vi "UniCyRO_Sim 2.vi"() -> ()   [LabVIEW 2012]
doc: "This VI starts and stops the environment simulator and serves as the master VI for your simulation code. Open and run this VI to display the environment simulator, or open the block diagram to view or modify simulation code."
uses:
  <vilib>/robotics/Simulator/Engine/ctl/Step Mode.ctl
  <vilib>/robotics/Simulator/Engine/ctl/Simulation Mode.ctl
  <vilib>/Simulation/Scripting/Companion Diagram/SimConfigNode/SimParams.ctl
  <vilib>/Simulation/Scripting/Companion Diagram/SimConfigNode/_simSolvers.ctl
  <vilib>/Simulation/Implementation/Shared/SIMSCR Execution Mode.ctl
  <vilib>/Platform/TimedLoop/XDataNode/timing_clust.ctl
  <vilib>/Platform/TimedLoop/XDataNode/nitl_modes.ctl
  <vilib>/Platform/TimedLoop/XDataNode/wakeup.ctl
  <vilib>/Simulation/Param Hierarchy/Typedefs/SIMPH Param Control Actions.ctl
  <vilib>/Simulation/Scripting/Editor Utilities/SIM subVI tag data.ctl
  <vilib>/Simulation/Scripting/Editor Utilities/SIM subVI execution type.ctl
  <vilib>/Simulation/Implementation/Shared/NILVSim_ParamChanged.vi
  <vilib>/Simulation/Implementation/Shared/NILVSim_FinishedLate.vi
  <vilib>/Simulation/Utility/Implementation/SIM Time.vi
  <vilib>/Simulation/Utility/Implementation/SIM Halt.vi
  <vilib>/Simulation/Implementation/Shared/SIM Fire Discrete SubVI.vi
  <vilib>/Simulation/Implementation/Shared/NILVSim_Manager.vi
  <vilib>/Simulation/Implementation/Shared/NILVSim_FinalizeModel.vi
  <vilib>/Simulation/Implementation/Shared/SIM Fire Discrete SubVI (Core).vi
  <vilib>/Simulation/Implementation/Shared/SIM Unbundle Sim Info.vi
  <vilib>/Utility/error.llb/Clear Errors.vi
  <vilib>/Simulation/Implementation/Shared/NILVSim_GetModelError.vi
  <vilib>/Simulation/Implementation/Shared/SIM Bundle Sim Info.vi
  <vilib>/Simulation/Implementation/Shared/SIMSH Read Queue.vi
  <vilib>/Simulation/Implementation/Shared/NILVSim_Initialize.vi
  Model/UniCyRO/Read Sensors.vi
  <vilib>/robotics/Simulator/Interface/Simulator References/Get Simulator Reference.vi
  <vilib>/robotics/Simulator/Interface/Simulator References/Get Joint Reference (Hinge).vi
  <vilib>/Simulation/Utility/Implementation/NILVSim Get Time and IsAcceptedStep.vi
  <vilib>/robotics/Simulator/Interface/Take Simulation Steps.vi
  <vilib>/Simulation/Scripting/Companion Diagram/SimConfigNode/SimDog.xnode
  Control Systems/PIDparallelController.vi
  Model/UniCyRO/UniCyRO_Host_Sim.lvclass
  <vilib>/Platform/TimedLoop/XDataNode/XDataNode.xnode
  <vilib>/Simulation/Implementation/XNodeFramework/SimXNode/SimX.xnode
  <vilib>/robotics/Simulator/NI_Robotics_Simulator.lvlib
  Model/UniCyRO/Set Motors.vi
  <resource>/objmgr/LVODE.rc
  <vilib>/Platform/TimedLoop/XDataNode/XDNodeRunTimeDep.lvlib
  <vilib>/Simulation/Implementation/Shared/NI_SIM_Implementation.lvlib
panel:
  out "floor(x/y)":dbl
  in  "Derivative time [s] (Td)":dbl=5.0
  in  "Integral time [s] (Ti)":dbl=1.0
  in  "Proportional Gain (Kc)":dbl=10.0
  in  "Accelerometer Gain":dbl(slide)=13.0 scale=0.0..100.0
  out "Waveform Chart":dbl(graph)
  in  "stop":bool
  in  "3D Visualization":refnum<vi>(3d-picture)
  in  "Gyro Motor ccw velocity (rad/s)":dbl(slide) scale=-20.0..20.0
  out "Drive Motor ccw velocity (rad/s)":dbl(slide) scale=-20.0..20.0
  in  "Torsion Motor ccw velocity (rad/s)":dbl(slide) scale=-20.0..20.0
  in  "manifest filename":string="UniCyRO_Sim.xml"
  # "Instructions:\n1. Run this VI.  \n2. The robot balances upright"
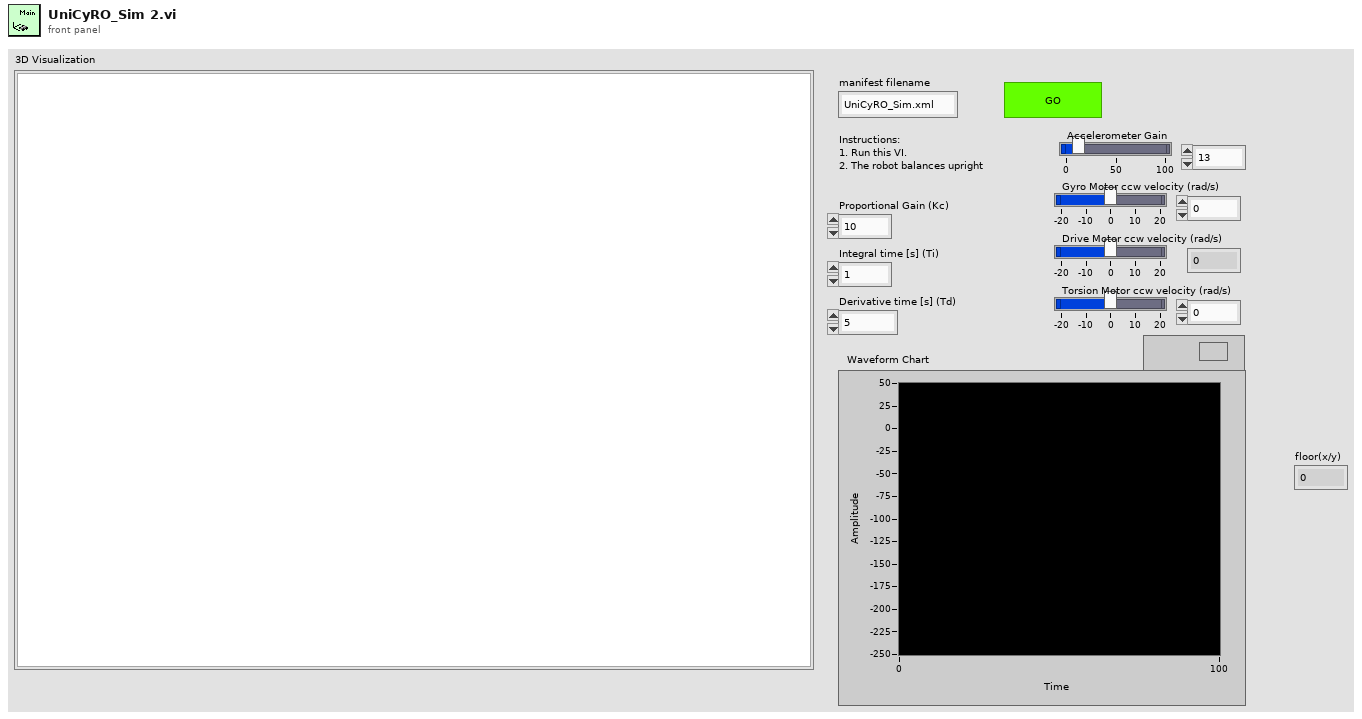
[diagram p1: front panel]
types:
  T1 = typedef "NI_Robotics_Simulator.lvlib/Simulation Mode.ctl" = u16
  T2 = typedef "NI_Robotics_Simulator.lvlib/Step Mode.ctl" = u16
  T3 = typedef "SIMSCR Execution Mode.ctl" = enum16{"Simulate to Completion", "Single Time-Step Simulation (Fixed Step Only)"}
  T4 = typedef "XDNodeRunTimeDep.lvlib/timing_clust.ctl" = cluster{"Expected End [f-1]":u64, "Actual End [f-1]":u64, "Finished Late? [f-1]":bool, "Expected End [i-1]":u64, "Actual End [i-1]":u64, "Finished Late? [i-1]":bool, "Expected Start [i]":u64, "Actual Start [i]":u64, "Expected Start [f]":u64, "Actual Start [f]":u64, "Source Name":string, "Structure Name":string, "Period":i64, "Deadline":i64, "Offset":i64, "Start":i64, "Priority":i32, "Timeout":i32, "Mode":T5, "Wakeup Reason":T6, "Error":errorcluster, "Source Type":string, "Secondary Source Type":string, "Global End Time":u64, "Global Start Time":u64, "Frame Duration":u64, "Iteration Duration":u64, "Assigned CPU":i32, "I/O Scan Engine Mode":u32}
  T5 = typedef "XDNodeRunTimeDep.lvlib/nitl_modes.ctl" = enum32{"No Change", "Process missed periods, maintain original phase", "Discard missed periods, maintain original phase", "Process missed periods, ignore original phase", "Discard missed periods, ignore original phase"}
  T6 = typedef "XDNodeRunTimeDep.lvlib/wakeup.ctl" = enum32{"Normal", "Aborted", "Asynchronous wakeup", "Timing source error", "Timed loop error", "Timeout"}
  T7 = typedef "SIMPH Param Control Actions.ctl" = enum16{"get params", "set params"}
  T8 = typedef "SIM subVI tag data.ctl" = cluster{"period":dbl, "skew":dbl, "Simulation execution type":T9}
  T9 = typedef "SIM subVI execution type.ctl" = enum16{"Function call", "Discrete", "Continuous", "Initialization only", "Final step only"}
  T10 = cluster{"SIMSH Sim Time":dbl, "Integral Gain - series.vi 2":cluster{"output":dbl}, "Integral Gain - series.vi 2 - SIMSH":cluster{"SIMSH Sim Time":dbl, "Select 2":cluster{"s? t:f":dbl}, "integral in gain?":bool, "Integrator":cluster{"output y(k)":dbl}, "Gain 2":cluster{"output":dbl}, "Select":cluster{"s? t:f":dbl}, "Equal To 0?":cluster{"x = 0?":bool}, "Reciprocal":cluster{"1/x":dbl}}, "SIM PID Derivative Gain.vi 2":cluster{"output":dbl}, "SIM PID Derivative Gain.vi 2 - SIMSH":cluster{"SIMSH Sim Time":dbl, "t 3":dbl, "Select 2":cluster{"s? t:f":dbl}, "Equal?":cluster{"x = y?":bool}, "Or":cluster{"x .or. y?":bool}, "Equal To 0?":cluster{"x = 0?":bool}}, "Gain 2":cluster{"output":dbl}, "Summation 2":cluster{"Result":dbl}}
  T11 = typedef "SimParams.ctl" = cluster{"Initial Time (s)":dbl, "Final Time (s)":dbl, "Step Size (s)":dbl, "ODE Solver":T12, "Minimum Step Size (s)":dbl, "Maximum Step Size (s)":dbl, "Relative Tolerance":dbl, "Absolute Tolerance":dbl, "Software Timing":bool, "Initial Step Size (s)":dbl, "Automatic Fixed Step Size?":bool, "Automatic Discrete Step Size?":bool, "Discrete Step Size (s)":dbl, "Calculate using Time Step":bool, "Solver Wired?":bool, "Prev.Frm.Expected End":u64, "Prev.Frm.Actual End":u64, "Prev.Frm.Finished Late?":bool, "Prev.Iter.Expected End":u64, "Prev.Iter.Actual End":u64, "Prev.Iter.Finished Late?":bool, "Expected Iteration Start":u64, "Actual Iteration Start":u64, "Expected Frame Start":u64, "Actual Frame Start":u64, "Source Name":string, "Name":string, "Period":i64, "Deadline":i64, "Offset":i64, "Start":i64, "Priority":i32, "Timeout":i32, "Processor":i32, "Mode":enum32{"No Change", "Process missed periods, maintain original phase", "Discard missed periods, maintain original phase", "Process missed periods, ignore original phase", "Discard missed periods, ignore original phase"}, "Wakeup reason":enum32{"Normal", "Aborted", "Asynchronous wakeup", "Timing source error", "Timed loop error", "Timeout"}, "Error":errorcluster, "Source Type":string, "Secondary Source Type":string, "Global End Time":u64, "Global Start Time":u64, "Full Solver Reset":bool, "Execution Mode":T3, "Nan/Inf Check":bool, "Custom Solver Library":string, "Solver Is Variable":bool, "custom solver name":string, "Signal Collection Decimation":u32}
  T12 = typedef "_simSolvers.ctl" = enum16{"Runge-Kutta 1 (Euler)", "Runge-Kutta 2", "Runge-Kutta 3", "Runge-Kutta 4", "Runge-Kutta 23 (variable)", "Runge-Kutta 45 (variable)", "BDF (variable)", "Adams-Moulton (variable)", "Rosenbrock (variable)", "Discrete States Only", "SDIRK 4 (variable)", "Radau 5 (variable)", "Radau 9 (variable)", "Radau 13 (variable)", "Radau [Variable Order] (variable)", "Gear's Method (variable)", "Linearizer", "State Query", "Trim Eval", "Custom Solver"}
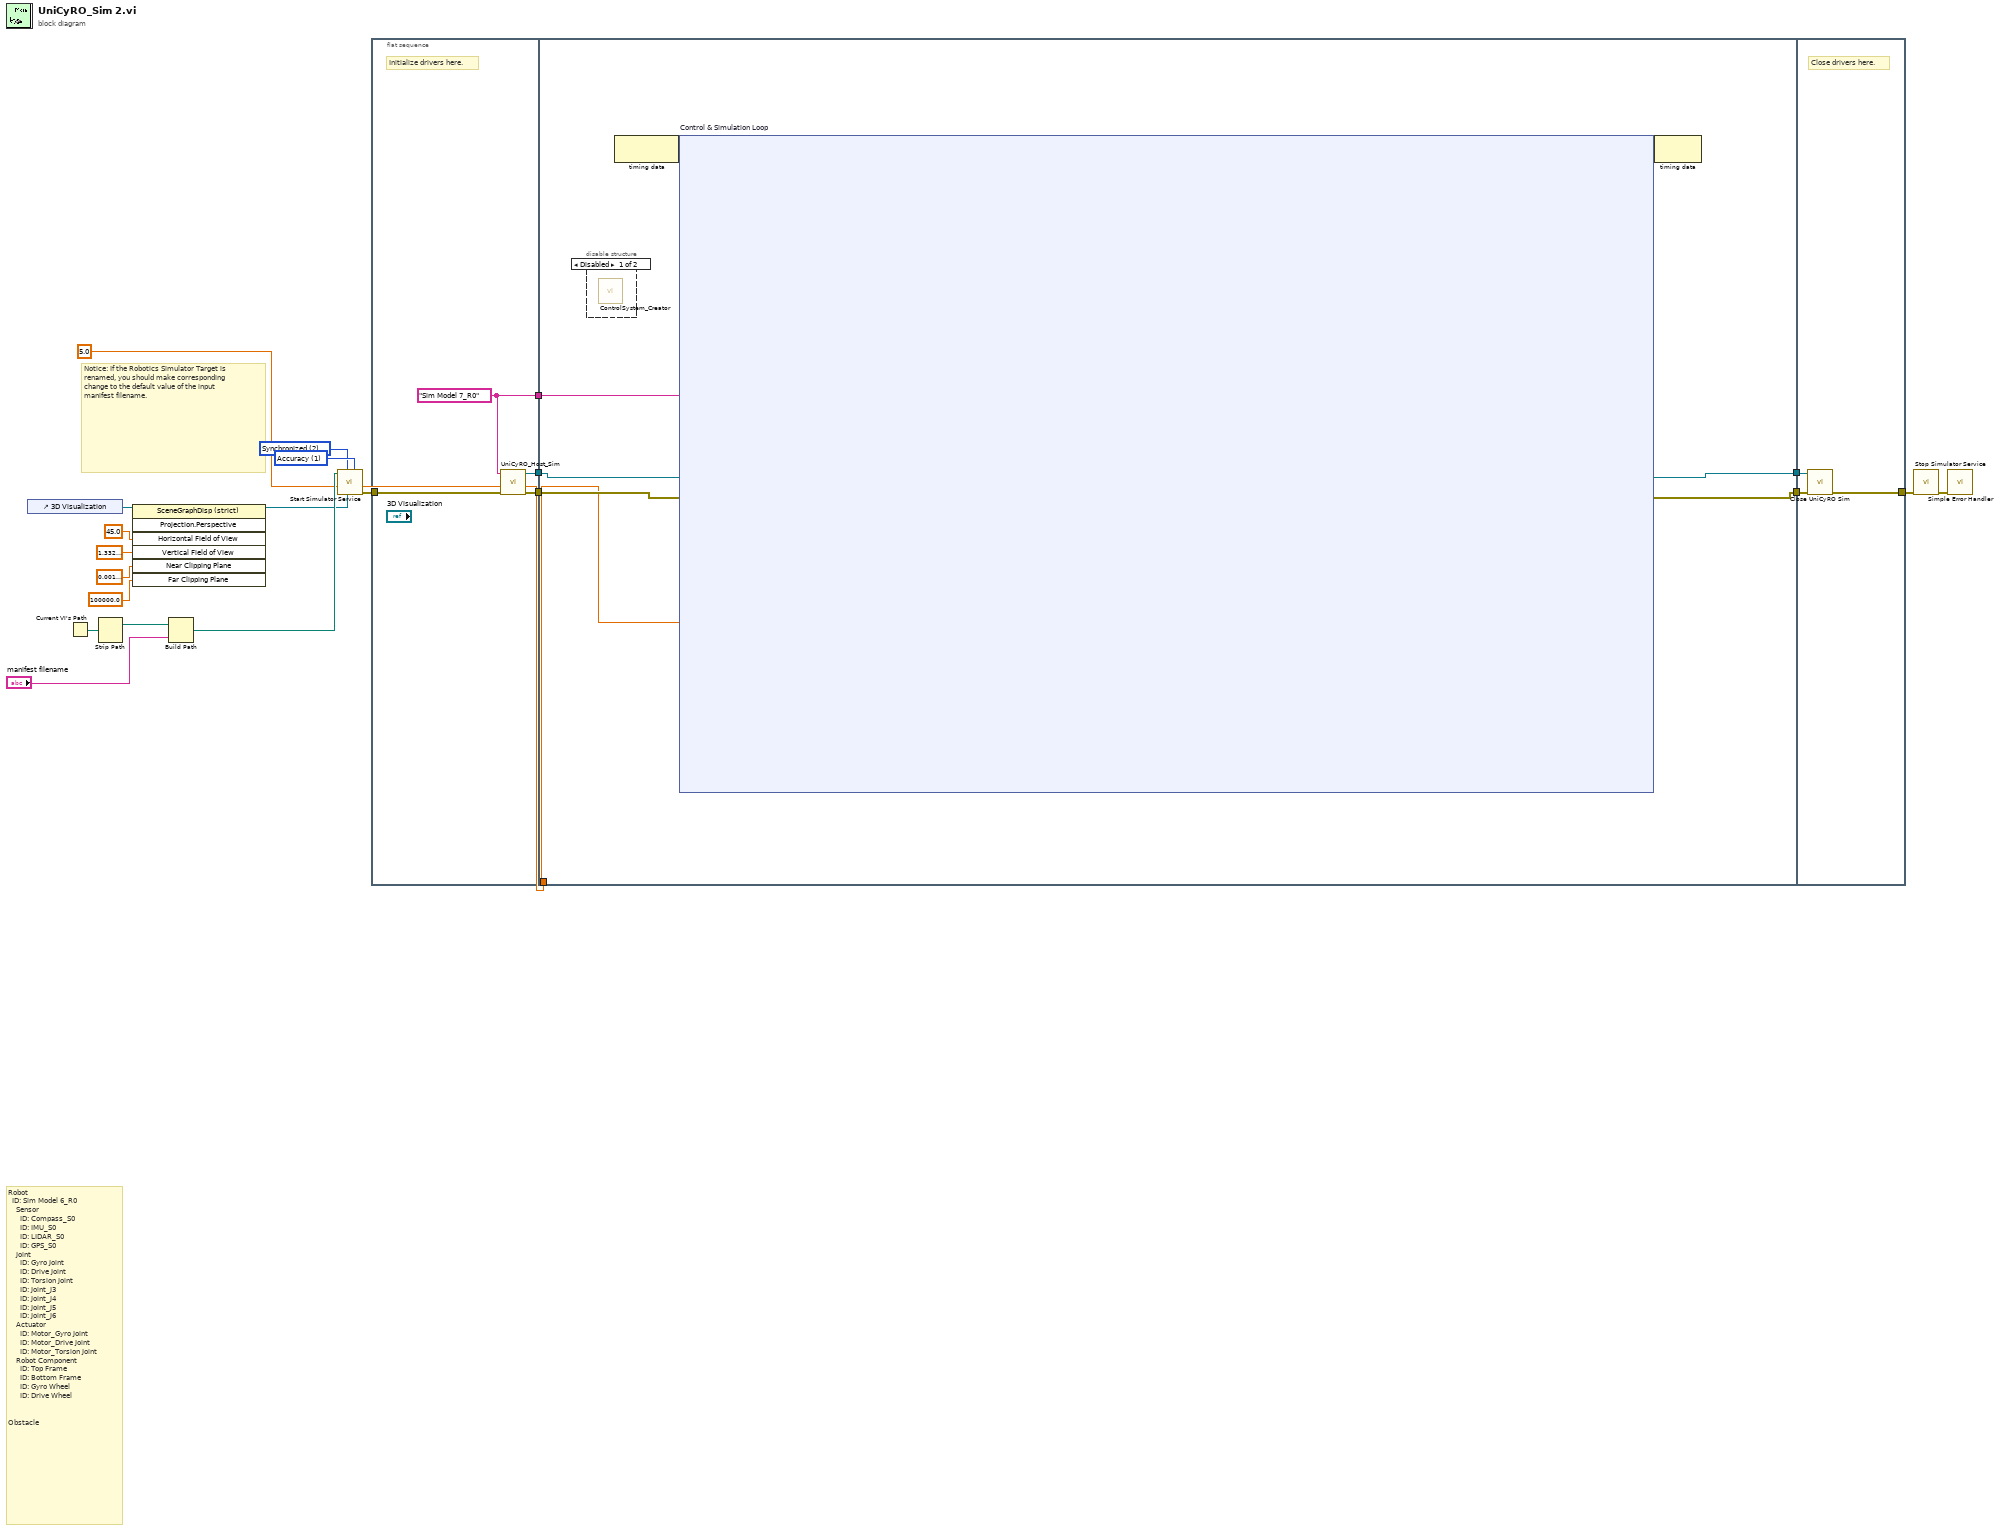
[diagram p0: block diagram]
diagram:
  w1 = T1 2 items=["Software Real-Time", "Free Running", "Synchronized"] ("timing mode")
  w5 = T2 1 items=["Performance", "Accuracy"] ("step mode")
  w2 = 5.0 ("stepsize(ms)")
  # "Robot\n\t\tID: Sim Model 6_R0\n\t\t\t\tSensor\n\t\t\t\t\t\tID: Compass_S0\n\t\t\t\t\t\tID: IMU_S0\n\t\t\t\t\t\tID: LIDAR_S0\n\t\t\t\t\t\tID: GPS_S0\n\t\t\t\tJoint\n\t\t\t\t\t\tID: Gyro Joint\n\t\t\t\t\t\tID: Drive Joint\n\t\t\t\t\t\tID: Torsion Joint\n\t\t\t\t\t\tID: Joint_J3\n\t\t\t\t\t\tID: Joint_J4\n\t\t\t\t\t\tID: Joint_J5\n\t\t\t\t\t\tID: Joint_J6\n\t\t\t\tActuator\n\t\t\t\t\t\tID: Motor_Gyro Joint\n\t\t\t\t\t\tID: Motor_Drive Joint\n\t\t\t\t\t\tID: Motor_Torsion Joint\n\t\t\t\tRobot Component\n\t\t\t\t\t\tID: Top Frame\n\t\t\t\t\t\tID: Bottom Frame\n\t\t\t\t\t\tID: Gyro Wheel\n\t\t\t\t\t\tID: Drive Wheel\n\n\nObstacle"
  # "Notice: If the Robotics Simulator Target is renamed, you should make corresponding change to the default value of the input manifest filename."
  n1 = control-ref of="3D Visualization"() -> (w9:refnum<vi>)
  n2 = Current VI's Path() -> (path=w20:path)
  n3 = Strip Path(path=w20) -> (stripped path=w19:path)  [unwired: 1 out]
  n4 = invoke on="Invoke Node" class="SceneGraphDisp (strict)" method="Projection.Perspective"(reference=w9, "Horizontal Field of View"=sgl 45.0 ("Field of View"), "Vertical Field of View"=sgl 1.333 ("Aspect Ratio"), "Near Clipping Plane"=sgl 0.001, "Far Clipping Plane"=sgl 100000.0) -> (reference out=w8:refnum<vi>)  [unwired: 2 in, 6 out]
  n5 = Build Path(base path=w19, name or relative path="manifest filename") -> (appended path=w18:path)
  n6 = call <vilib>:"Start Simulator Service.vi"("step mode"=w5, "3D picture refnum"=w8, "timing mode"=w1, "step size (ms)"=w2, "manifest file"=w18) -> ("error out"=w4:errorcluster)  [unwired: 6 in]
  n7 = flat-sequence {
    tunnel: [w25] -> w15
    tunnel: [w24] -> w14
    tunnel: [w23] -> w7
    tunnel: w4 -> [w22]
    tunnel: w15 -> [w29]
    tunnel: w14 -> [w30]
    tunnel: [w28] -> w13
    tunnel: w7 -> [w31]
    tunnel: [w27] -> w3
    tunnel: w2 -> [w26]
    tunnel: [w521] -> w21
    tunnel: w13 -> [w523]
    tunnel: w3 -> [w522]
    frame #0 {
      w23 = "Sim Model 7_R0"
      # "Initialize drivers here."
      n8 = call "UniCyRO_Host_Sim"("error in (no error)"=w22, "robot ID"=w23) -> ("error out"=w25:errorcluster, "UniCyRO_Host_Sim out"=w24:refnum<class "UniCyRO_Host_Sim.lvclass">)  [unwired: 8 in]
    }
    frame #1 {
      n9 = disable-structure shown="Disabled" {
        frame Disabled {
          n10 = call "ControlSystem_Creator.vi"() -> ()  [unwired: 9 in, 7 out]
        }
        frame Enabled {
        }
      }
      n11 = node-c288() -> (w33:variant)  [unwired: 1 in]
      n12 = node-c254 "Control & Simulation Loop"(w33, w31, w30, w29, w26) -> (w32:variant, w28:refnum<class "UniCyRO_Host_Sim.lvclass">, w27:errorcluster)
      n13 = node-c288(w32) -> ()  [unwired: 1 out]
    }
    frame #2 {
      # "Close drivers here."
      n14 = call "Close UniCyRO Sim.vi"("error in (no error)"=w522, "UniCyRO_Host_Sim in"=w523) -> ("error out"=w521:errorcluster)  [unwired: 9 in]
    }
  }
  n15 = call <vilib>:"Stop Simulator Service.vi"("error in (no error)"=w21) -> ("error out"=w16:errorcluster)  [unwired: 10 in]
  n16 = call <vilib>:"Simple Error Handler.vi"("error in (no error)"=w16) -> ()  [unwired: 4 in, 5 out]
